vi "8-Byte Array To MAC.vi"(1 "Byte Array":u8[](array[numeric])) -> (0 "MAC (hexdot string)":string)   [LabVIEW 2024]
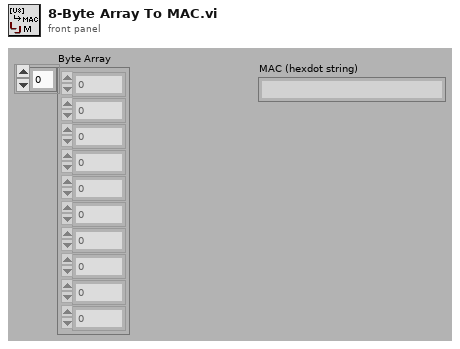
[diagram p1: front panel]
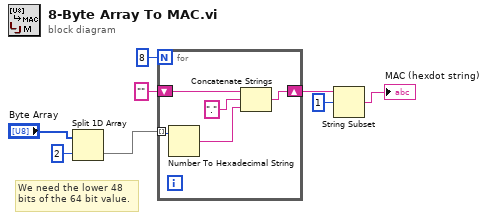
[diagram p0: block diagram]
diagram:
  # "We need the lower 48\nbits of the 64 bit value."
  n1 = Split 1D Array(array="Byte Array", index=2) -> (second subarray=w1:u8[])  [unwired: 1 out]
  n2 = for {
    N: 8 -> [_]
    tunnel: w1 -> [w13] mode=indexing
    shift-right: [w11] -> w5
    shift-left: "" -> [w10]
    n3 = Number To Hexadecimal String(2:w13) -> (0:w9:string)  [unwired: 1 in]
    n4 = Concatenate Strings(w10, "." ("string"), w9) -> (w11:string)
  }
  n5 = String Subset(string=w5, offset (0)=1) -> (substring=→"MAC (hexdot string)":string)  [unwired: 1 in]
